vi "ABR-Init Hardware.vi"(0 "Stimulus":T2={"Ear"=enum."Left", "Start (dB)"=20, "Waveform"=enum."TONE PIP", "Stop (dB)"=80, "Frequency (kHz)"=16.0, "Step (dB)"=5, "Rep rate (/sec)"=30.0, "Alternate Polarity"=FALSE} {"Frequency (kHz)" format="%.2f"; "Start (dB)" step=5}, 1 "CAP or ABR":u16(ring)=1 items=["CAP", "ABR"], 9 "Hidden":T3={"AI Samp Rate Hz"=25000.0, "AO Samp Rate Hz"=100000.0, "Duration (ms)"=5.0, "Ramp (ms)"=0.5, "Click width (us)"=0.0, "ITI"=enum."Rate", "Save raw"=FALSE}, 11 "error in (no error)":errorcluster) -> (4 "AO Channels":i32[](array[numeric]), 6 "Runtime":T1, 8 "Coerced rep rate":dbl, 15 "error out":errorcluster)   [LabVIEW 2020]
uses:
  TypeDefs/ABR-Hidden Params.ctl
  TypeDefs/ABR-Stimulus.ctl
  TypeDefs/ABR-Runtime Data.ctl
  epl-vi-lib/Connection VIs/Type Defs/Input sources.ctl
  epl-vi-lib/Connection VIs/Type Defs/Output sources.ctl
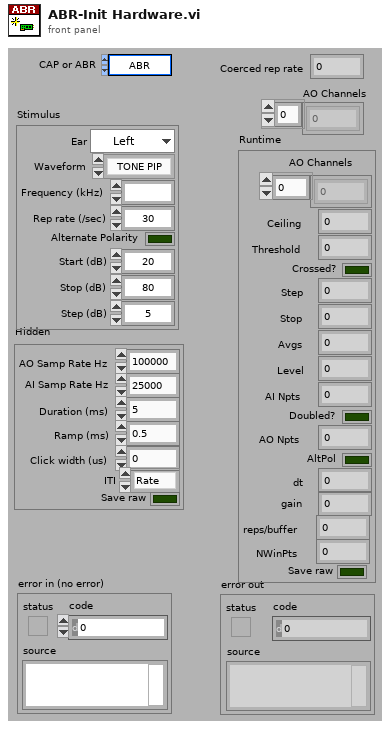
[diagram p1: front panel]
types:
  T1 = typedef "ABR-Runtime Data.ctl" = cluster{"AO Channels":i32[], "Ceiling":dbl, "Threshold":dbl, "Crossed?":bool, "Step":dbl, "Stop":i32, "Avgs":i32, "Level":dbl, "AI Npts":i32, "Doubled?":bool, "AO Npts":i32, "AltPol":bool, "dt":dbl, "gain":dbl, "reps/buffer":i32, "NWinPts":i32, "Save raw":bool}
  T2 = typedef "ABR-Stimulus.ctl" = cluster{"Ear":enum16{"Right", "Left", "Bone"}, "Start (dB)":i32, "Waveform":enum16{"TONE PIP", "CLICK"}, "Stop (dB)":i32, "Frequency (kHz)":ext, "Step (dB)":i32, "Rep rate (/sec)":dbl, "Alternate Polarity":bool}
  T3 = typedef "ABR-Hidden Params.ctl" = cluster{"AI Samp Rate Hz":dbl, "AO Samp Rate Hz":dbl, "Duration (ms)":dbl, "Ramp (ms)":dbl, "Click width (us)":dbl, "ITI":enum16{"Rate", "Interval"}, "Save raw":bool}
  T4 = typedef "Input sources.ctl" = u16
  T5 = typedef "Output sources.ctl" = u16
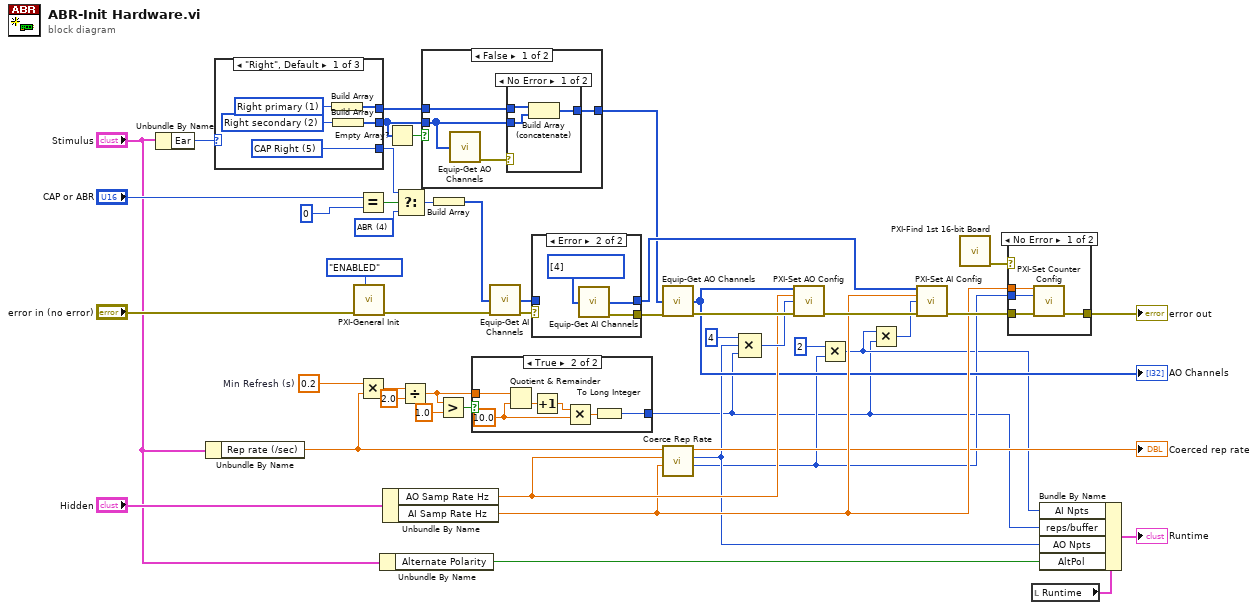
[diagram p0: block diagram]
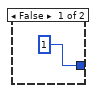
[diagram p5: hidden frame]
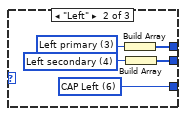
[diagram p7: hidden frame]
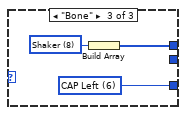
[diagram p8: hidden frame]
diagram:
  w11 = 0.2  # Min Refresh (s)
  w34 = T4 4 items=["--unused--", "Probe Mic Right", "Probe Mic Left", "Cal Mic", "ABR", "CAP Right", "CAP Left", "Startle piezo", "Temperature", "Heart rate"] ("Ring")
  n1 = Unbundle By Name("Stimulus") -> ("Ear"=w27:enum16{"Right", "Left", "Bone"})
  n2 = Unbundle By Name("Stimulus") -> ("Rep rate (/sec)"=w10:dbl)
  n3 = case shown="\"Right\", Default" w27 {
    tunnel: [w51 w56 w59] -> w5
    tunnel: [w53 w58 w61] -> w32
    tunnel: [w49 w54 _] -> w4
    frame "Right", Default {
      w50 = T5 2 items=["--unused--", "Right primary", "Right secondary", "Left primary", "Left secondary", "Shocks", "Startle", "Background"] ("Ring")
      w53 = T4 5 items=["--unused--", "Probe Mic Right", "Probe Mic Left", "Cal Mic", "ABR", "CAP Right", "CAP Left", "Startle piezo", "Temperature", "Heart rate"] ("Ring")
      w52 = T5 1 items=["--unused--", "Right primary", "Right secondary", "Left primary", "Left secondary", "Shocks", "Startle", "Background"] ("Ring")
      n4 = Build Array(w52) -> (w51:T5[])
      n5 = Build Array(w50) -> (w49:T5[])
    }
    frame "Left" {
      w55 = T5 4 items=["--unused--", "Right primary", "Right secondary", "Left primary", "Left secondary", "Shocks", "Startle", "Background", "Shaker"] ("Ring")
      w58 = T4 6 items=["--unused--", "Probe Mic Right", "Probe Mic Left", "Cal Mic", "ABR", "CAP Right", "CAP Left", "Startle piezo", "Temperature", "Heart rate"] ("Ring")
      w57 = T5 3 items=["--unused--", "Right primary", "Right secondary", "Left primary", "Left secondary", "Shocks", "Startle", "Background"] ("Ring")
      n6 = Build Array(w57) -> (w56:T5[])
      n7 = Build Array(w55) -> (w54:T5[])
    }
    frame "Bone" {
      w60 = T5 8 items=["--unused--", "Right primary", "Right secondary", "Left primary", "Left secondary", "Shocks", "Startle", "Background", "Shaker", "Blue laser"] ("Output sources")
      w61 = T4 6 items=["--unused--", "Probe Mic Right", "Probe Mic Left", "Cal Mic", "ABR", "CAP Right", "CAP Left", "Startle piezo", "Temperature", "Heart rate"] ("Ring")
      n8 = Build Array(w60) -> (w59:T5[])
    }
  }
  n9 = call "PXI-General Init.vi"("Double Buffer Mode"=enum32{"OFF", "ENABLED", "FORCED"}."ENABLED", "error in (no error)"="error in (no error)") -> ("error out"=w45:errorcluster)  [unwired: 9 in]
  n10 = Equal?(x="CAP or ABR", y=u16 0) -> (x = y?=w37:bool)
  n11 = Multiply(x=w11, y=w10) -> (x*y=w12:dbl)
  n12 = Unbundle By Name("Stimulus") -> ("Alternate Polarity"=w17:bool)
  n13 = Unbundle By Name("Hidden") -> ("AO Samp Rate Hz"=w39:dbl, "AI Samp Rate Hz"=w38:dbl)
  n14 = Empty Array?(array=w4) -> (empty?=w3:bool)
  n15 = Select(t=w32, s=w37, f=w34) -> (s? t:f=w31:T4)
  n16 = Divide(x=w12, y=2.0) -> (x/y=w15:dbl)
  n17 = case shown="False" w3 {
    tunnel: w5 -> [w65 w70]
    tunnel: w4 -> [w63 _]
    tunnel: [w62 w70] -> w2
    frame False {
      n18 = call "Equip-Get AO Channels.vi"("Outputs"=w63) -> ("error out"=w64:errorcluster)  [unwired: 13 in, 1 out]
      n19 = case shown="No Error" w64 {
        tunnel: w65 -> [w68 w69]
        tunnel: w63 -> [w67 _]
        tunnel: [w66 w69] -> w62
        frame No Error {
          n20 = Build Array (concatenate)(w68, w67) -> (w66:T5[])
        }
        frame Error {
        }
      }
    }
    frame True {
    }
  }
  n21 = Build Array(w31) -> (w30:T4[])
  n22 = Greater?(x=w15, y=1.0) -> (0:w14:bool)
  n23 = case shown="True" w14 {
    tunnel: w15 -> [_ w77]
    tunnel: [1 w73] -> w6
    frame False {
    }
    frame True {
      w76 = 10.0 ("y")
      n24 = Quotient & Remainder(x=w77, y=w76) -> (floor(x/y)=w74:dbl)  [unwired: 1 out]
      n25 = Increment(x=w74) -> (x+1=w72:dbl)
      n26 = Multiply(x=w72, y=w76) -> (x*y=w75:dbl)
      n27 = To Long Integer(number=w75) -> (32bit integer=w73:i32)
    }
  }
  n28 = call "Equip-Get AI Channels.vi"("Inputs"=w30, "error in (no error)"=w45) -> ("AI Channels"=w23:i32[], "error out"=w24:errorcluster)  [unwired: 12 in]
  n29 = case shown="Error" w24 {
    selector: w24 -> [w78 _]
    tunnel: [w79 w80] -> w21
    tunnel: w23 -> [w79 _]
    tunnel: [w78 w81] -> w22
    frame No Error {
    }
    frame Error {
      w82 = T4[] [4] items=["--unused--", "Probe Mic Right", "Probe Mic Left", "Cal Mic", "ABR", "CAP Right", "CAP Left", "Startle piezo", "Temperature", "Heart rate"]
      n30 = call "Equip-Get AI Channels.vi"("Inputs"=w82) -> ("AI Channels"=w80:i32[], "error out"=w81:errorcluster)  [unwired: 13 in]
    }
  }
  n31 = call "Equip-Get AO Channels.vi"("Outputs"=w2, "error in (no error)"=w22) -> ("AO Channels"=w28:i32[], "error out"=w44:errorcluster)  [unwired: 12 in]
  "AO Channels" <- w28
  n32 = call "Coerce Rep Rate.vi"("AI sampling rate (Hz)"=w38, "AO sampling rate (Hz)"=w39, "Rep rate (Hz)"=w10) -> ("AI npts"=w9:i32, "AO npts"=w25:i32, "Coerced rep rate (Hz)"=→"Coerced rep rate":dbl)  [unwired: 5 in, 1 out]
  n33 = Compound Arithmetic op=MULTIPLY(4 ("x"), w25, w6) -> (w43:i32)
  n34 = call "PXI-Set AO Config.vi"("AO Channels"=w28, "Sampling Rate (Hz)"=w39, "Buffer Size"=w43, "error in (no error)"=w44) -> ("error out"=w42:errorcluster)  [unwired: 11 in]
  n35 = Multiply(x=2, y=w9) -> (x*y=w8:i32)
  n36 = Multiply(x=w8, y=w6) -> (x*y=w7:i32)
  n37 = call "PXI-Set AI Config.vi"("AI Channels"=w21, "Sampling Rate (Hz)"=w38, "Buffer Size"=w7, "error in (no error)"=w42) -> ("error out"=w41:errorcluster)  [unwired: 11 in]
  n38 = call "PXI-Find 1st 16-bit Board.vi"() -> ("error out"=w1:errorcluster)  [unwired: 9 in, 2 out]
  n39 = case shown="No Error" w1 {
    tunnel: w41 -> [w86 w87]
    tunnel: w38 -> [w85 _]
    tunnel: [w84 w87] -> w29
    tunnel: w9 -> [w83 _]
    frame No Error {
      n40 = call "PXI-Set Counter Config.vi"("AI Sampling Rate (Hz)"=w85, "Num AI Pts"=w83, "error in (no error)"=w86) -> ("error out"=w84:errorcluster)  [unwired: 12 in]
    }
    frame Error {
    }
  }
  "error out" <- w29
  n41 = local read "Runtime"() -> (w20:T1)
  n42 = Bundle By Name(cluster=w20, "AI Npts"=w8, "reps/buffer"=w6, "AO Npts"=w25, "AltPol"=w17) -> (→"Runtime":T1)
